vi "GetFontsList.vi"(5 "error in (no error)":errorcluster) -> (15 "Fonts Installed":string[](array[string]), 19 "error out":errorcluster)   [LabVIEW 2017, in "G#IDE.lvlib" / "IconLib.lvlib"]
uses:
  <resource>/Framework/Providers/AddQ/G#IDE/support/IconLib/IconLib.lvlib
  <vilib>/registry/registry.llb/Registry RtKey.ctl
  <vilib>/registry/registry.llb/Registry SAM.ctl
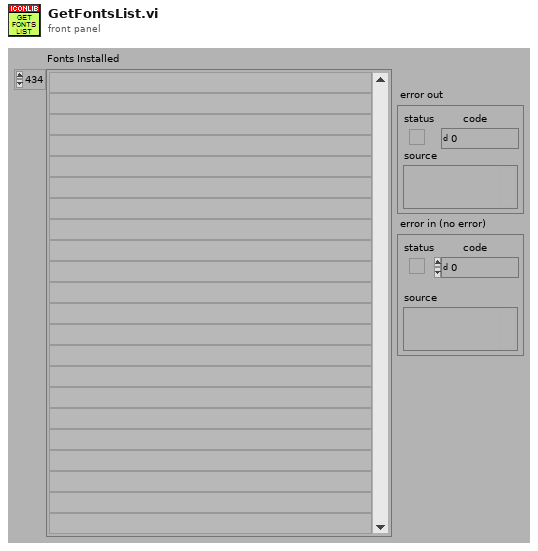
[diagram p1: front panel]
types:
  T1 = typedef "Registry SAM.ctl" = enum32{"KEY_QUERY_VALUE", "KEY_SET_VALUE", "KEY_CREATE_SUB_KEY", "KEY_ENUMERATE_SUB_KEYS", "KEY_NOTIFY", "KEY_CREATE_LINK", "KEY_READ", "KEY_WRITE", "KEY_ALL_ACCESS", "KEY_READ | KEY_WRITE"}
  T2 = typedef "Registry RtKey.ctl" = enum32{"HKEY_CLASSES_ROOT", "HKEY_CURRENT_USER", "HKEY_LOCAL_MACHINE", "HKEY_USERS", "HKEY_PERFORMANCE_DATA", "HKEY_CURRENT_CONFIG", "HKEY_DYN_DATA"}
  T3 = typedef "Registry refnum.ctl" = refnum<k1>
  T4 = cluster{"numValues":i32, "maxValueNameLen":i32, "maxValueDataLen":i32}
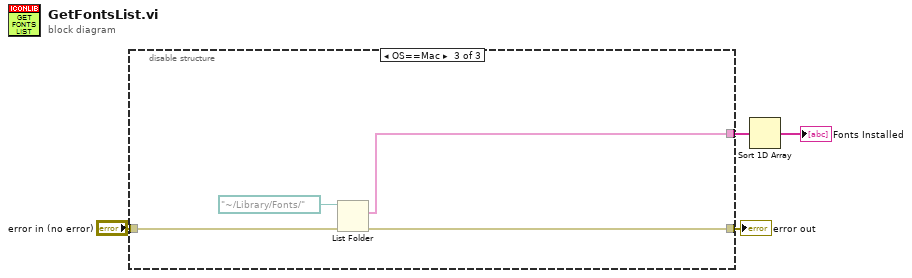
[diagram p0: block diagram]
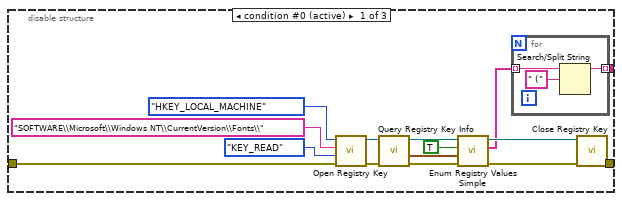
[diagram p2: hidden frame]
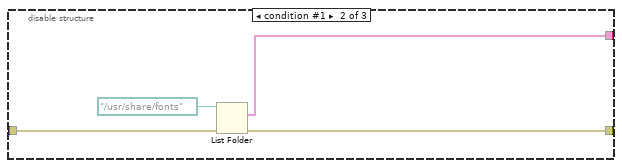
[diagram p3: hidden frame]
diagram:
  n1 = disable-structure shown="OS==Mac" {
    disable-tunnel: [w17 w24 w28] -> w4
    disable-tunnel: [w6 w23 w27] -> w3
    disable-tunnel: "error in (no error)" -> [w5 w25 w29]
    frame condition #0 (active) {
      n2 = call <vilib>:"Open Registry Key.vi"("error in (no error)"=w5, "security access mask (KEY_READ | KEY_WRITE)"=Registry_SAM."KEY_READ", "subkey"="SOFTWARE\\Microsoft\\Windows NT\\CurrentVersion\\Fonts\\", "root key (HKEY_LOCAL_MACHINE)"=Registry_RtKey."HKEY_LOCAL_MACHINE") -> ("error out"=w15:errorcluster, "refnum out"=w16:T3)  [unwired: 6 in]
      n3 = call <vilib>:"Query Registry Key Info.vi"("error in (no error)"=w15, "refnum"=w16) -> ("error out"=w12:errorcluster, "value info"=w9:T4, "refnum out"=w13:T3)  [unwired: 5 in, 2 out]
      n4 = call <vilib>:"Enum Registry Values Simple.vi"("error in (no error)"=w12, "value info"=w9, "retrieve data? (F)"=TRUE, "refnum"=w13) -> ("error out"=w11:errorcluster, "values"=w7:string[], "refnum out"=w10:T3)  [unwired: 2 in, 3 out]
      n5 = for {
        tunnel: w7 -> [w22] mode=indexing
        tunnel: [w20] -> w6 mode=indexing
        n6 = Search/Split String(string=w22, search string/char (-)=" (") -> (substring before match=w20:string)  [unwired: 1 in, 2 out]
      }
      n7 = call <vilib>:"Close Registry Key.vi"("error in (no error)"=w11, "refnum"=w10) -> ("error out"=w17:errorcluster)  [unwired: 5 in]
    }
    frame condition #1 {
      n8 = List Folder(path=path "/usr/share/fonts", error in=w25) -> (filenames=w23:string[], error out=w24:errorcluster)  [unwired: 2 in, 2 out]
    }
    frame condition #2 {
      n9 = List Folder(path=path "~/Library/Fonts/", error in=w29) -> (filenames=w27:string[], error out=w28:errorcluster)  [unwired: 2 in, 2 out]
    }
  }
  "error out" <- w4
  n10 = Sort 1D Array(array=w3) -> (sorted array=→"Fonts Installed":string[])
